vi "ISM Release Pump.vi"(8 "error in (no error)":errorcluster, 11 "Pump Number In":i32) -> (0 "error out":errorcluster, 3 "Pump Number Out":i32)   [LabVIEW 2018, in "Ismatec 4308.lvlib"]
uses:
  Ismatec 4308.lvlib
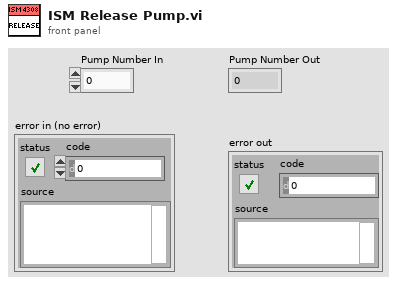
[diagram p1: front panel]
types:
  T1 = cluster{"Busy":bool, "ChannelCnt":dbl, "Initialized":bool, "Current Channel":dbl, "Initialized Channels":dbl[]}[]
  T2 = cluster{"Busy":bool, "ChannelCnt":dbl, "Initialized":bool, "Current Channel":dbl, "Initialized Channels":dbl[]}
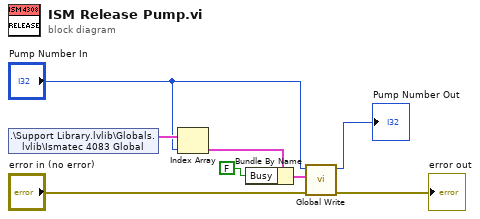
[diagram p0: block diagram]
diagram:
  n1 = shared-variable ".\\Support Library.lvlib\\Globals.lvlib\\Ismatec 4083 Global"() -> (w7:T1)  [unwired: 1 in, 1 out]
  n2 = Index Array(array=w7, index="Pump Number In") -> (element=w6:T2)
  n3 = Bundle By Name(cluster=w6, "Busy"=FALSE) -> (w5:T2)
  n4 = call "Global Write.vi"("error in (no error)"="error in (no error)", "Incoming Cluster"=w5, "Pump Number In"="Pump Number In") -> ("error out"=→"error out":errorcluster, "Pump Number Out"=→"Pump Number Out":i32)  [unwired: 7 in]
